vi "Set Engine Scan Rate.vi"(8 "error in (no error)":errorcluster, 10 "scan period (uSec)":u32=10000, 11 "references in":T1) -> (0 "error out":errorcluster, 3 "references out":T1)   [LabVIEW 2013, in "Scan Engine configuration.lvclass"]
uses:
  Scan Engine configuration.lvclass
  <vilib>/NI/DCAF Table API/Table Manager/object ref.ctl
  <vilib>/NI/DCAF/Tag Editor Core/Configuration Editor/Classes/Engine Parent/Engine Parent Editor Node.lvclass
  <vilib>/NI/DCAF/Tag Editor Core/Configuration Editor/Classes/Module editor node/module editor node.lvclass
  <vilib>/NI/DCAF/Tag Editor Core/Configuration Editor/Classes/Module editor node/Read Module Configuration.vi
  <vilib>/NI/DCAF/Tag Editor Core/Configuration Editor/Classes/Module editor node/Write Module Configuration.vi
  <vilib>/NI/Tag Bus Module Framework/module configuration/TBM module configuration.lvclass
  <vilib>/NI/DCAF Table API/Table Manager/Table Manager.lvclass
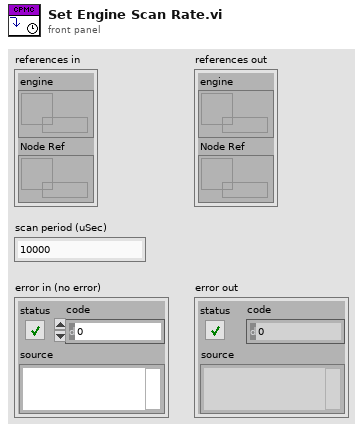
[diagram p1: front panel]
types:
  T1 = typedef "Table Manager.lvlib/Table Manager.lvclass/object ref.ctl" = cluster{"engine":refnum<data-value>, "Node Ref":refnum<data-value>}
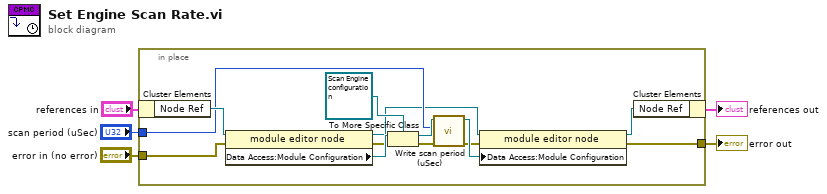
[diagram p0: block diagram]
diagram:
  n1 = in-place {
    in-place-border: "scan period (uSec)" -> [w14]
    in-place-border: "error in (no error)" -> [w10]
    in-place-border: [w6] -> w2
    n2 = in-place-cluster #1("references in") -> ("Node Ref"=w17:refnum<data-value>)
    n3 = property class="module editor node"(reference=w17, error in=w10) -> (reference out=w12:refnum<data-value>, error out=w9:errorcluster, "Data Access:Module Configuration"=w16:refnum<class "TBM module configuration.lvclass">)
    n4 = To More Specific Class(target class=refnum<class "Scan Engine configuration.lvclass"> refnum ("Scan Engine configuration"), reference=w16, error in=w9) -> (specific class reference=w15:refnum<class "Scan Engine configuration.lvclass">, error out=w8:errorcluster)
    n5 = call-dynamic "Write scan period (uSec).vi"("error in (no error)"=w8, "scan period (uSec)"=w14, "Scan Engine configuration1 in"=w15) -> ("error out"=w7:errorcluster, "Scan Engine configuration1 out"=w13:refnum<class "Scan Engine configuration.lvclass">)  [unwired: 7 in]
    n6 = property class="module editor node"(reference=w12, error in=w7, "Data Access:Module Configuration"=w13) -> (reference out=w11:refnum<data-value>, error out=w6:errorcluster)
    n7 = in-place-cluster #1("Node Ref"=w11) -> (→"references out":T1)
  }
  "error out" <- w2
